vi "SimulatoreStep.vi"() -> ()   [LabVIEW 2019]
doc: "Simulatore Step dei Test:\n\n1. Seleziona la postazione con la data di partenza (opzionale)\n2. Seleziona il Test che vuoi eseguire\n3. Avvia la simulazione e verifica il successo degli Step"
uses:
  ByteGSAPIBase/ByteGSAPIBase.lvclass
  TypeDef/StepSimulationInfo.ctl
  TypeDef/ProcessStatus.ctl
  TypeDef/SimulatoreStates.ctl
  ByteGSAPIBase/TypeDef/Step.ctl
  ByteGSAPIBase/TypeDef/Asset.ctl
  ByteGSAPIBase/TypeDef/Test.ctl
  <vilib>/numeric/Random Number (Range) U64.vi
  <vilib>/numeric/sub_Random U32.vi
panel:
  out "Title":string
  out "Status Control":T2
  out "Waveform Chart":cluster{"Time Elapsed":dbl, dbl}(graph)
  out "Step Info List":T3[](array[typedef])
  in  "Step simulation":bool
  out "Infos":string
  in  "Inizia Test":bool
  in  "Select Test":i32(ring) items=["Test Endurance"=35, "Test Endurance"=36, "Test su Statore H100 dia 65"=29, "Test su Statore H100 dia 65"=31, "Test Endurance"=34, "Test su Statore H100 dia 65"=30, "Effettuare prova sul banco Labview su campione ABC"=40, "Test doppio carico per freni 50Nm/12rpm"=26, "Test su Statore H100 dia 65"=27, "Test su Statore H100 dia 65"=28, "Test su Statore H100 dia 65"=32]
  in  "ByteGSAPIBase in":refnum<class "ByteGSAPIBase.lvclass">
  in  "Exit":bool
  in  "Home":bool
  in  "Ottieni Test Per Postazione":bool
  in  "Starting Date":timestamp format="%<%x>T"
  in  "Workstation":enum16{"POST 1"}(ring)
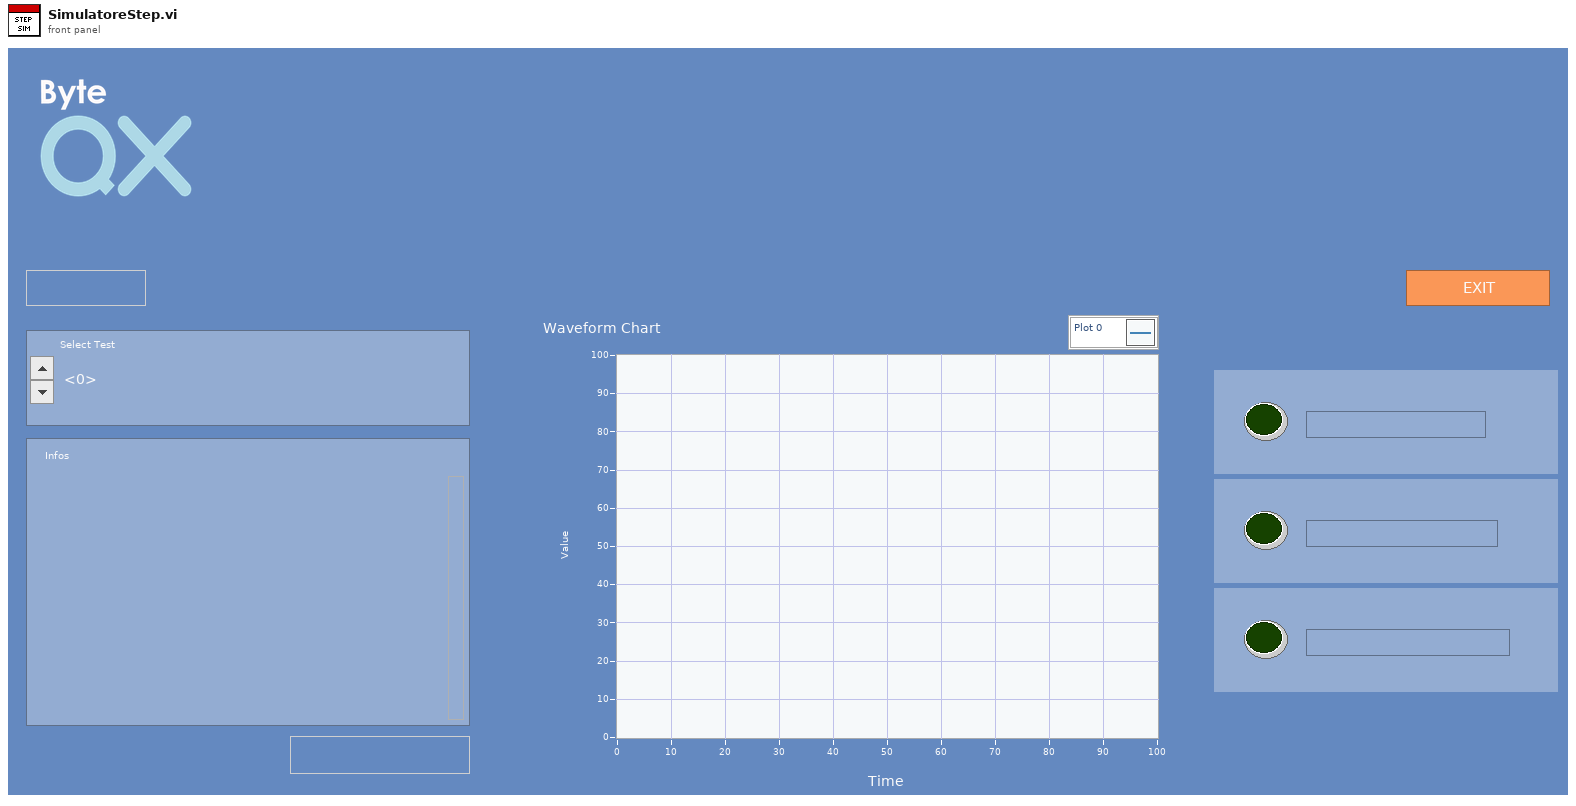
[diagram p1: front panel]
types:
  T1 = typedef "ProcessStatus.ctl" = cluster{"Active":bool, "Process":string}
  T2 = cluster{"Cluster":T1, "Cluster 2":T1, "Cluster 3":T1}
  T3 = typedef "StepSimulationInfo.ctl" = cluster{"Description":string, "Value":dbl, "Outcome":string, "Time Elapsed":dbl, "id":dbl, "Color Box":u32}
  T4 = typedef "SimulatoreStates.ctl" = enum16{"Initialize", "Idle", "GetLimsTestsForBench", "GetLimsTestSteps", "Simulation Start", "WaitForLigths"}
  T5 = typedef "ByteGSWebAPI.lvlib/ByteGSAPIBase.lvclass/Test.ctl" = cluster{"titolo":string, "descrizione":string, "statoprova":string, "assets":T6[], "id":i32, "data_apertura_prova":timestamp}
  T6 = typedef "ByteGSWebAPI.lvlib/ByteGSAPIBase.lvclass/Asset.ctl" = cluster{"descrizione":string, "slug":string, "id":i32}
  T7 = typedef "ByteGSWebAPI.lvlib/ByteGSAPIBase.lvclass/Step.ctl" = cluster{"id":i32, "descrizione":string, "prova":string, "assets":T6[], "criterio_accettazione":string, "valore_criterio_accettazione_max":dbl, "valore_criterio_accettazione_min":dbl, "udm_criterio_accettazione":string, "duration_prova":string, "udm_duration_prova":string, "valore_prova":dbl, "ordine":i32, "user":i32, "link_automation":string, "instruction_automation":string, "data_completamento_checklist":timestamp, "outcome":bool}
  T8 = cluster{"ByteGSAPIBase in":refnum<class "ByteGSAPIBase.lvclass">, "Array dei Test":T5[], "Steps Array":T7[], "Step Info List":T3[], "index":i32, "Previus":T4, "Infos":string, "State":T4, "Status Control":cluster{"Cluster":T1, "Cluster 2":T1, "Cluster 3":T1}, "light position":i32}
  T9 = cluster{"Workstation":refnum<vi>, "Starting Date":refnum<vi>, "Ottieni Test Per Postazione":refnum<vi>, "Infos":refnum<vi>, "Inizia Test":refnum<vi>, "Select Test":refnum<vi>, "Step Info List":refnum<vi>, "Step simulation":refnum<vi>, "Waveform Chart":refnum<vi>, "Status Control":refnum<vi>, "Title":refnum<vi>}
  T10 = enum8{"Enabled", "Disabled", "Disabled and Grayed Out"}
  T11 = cluster{"Workstation":enum16{"POST 1"}, "Starting Date":timestamp, "Select Test":i32}
  T12 = typedef "ByteGSWebAPI.lvlib/ByteGSAPIBase.lvclass/UpdateLimsTestStepData.ctl" = cluster{"outcome":bool, "data_completamento_checklist":timestamp, "udm_duration_prova":string, "valore_prova":dbl, "link_automation":string, "instruction_automation":string, "duration_prova":string}
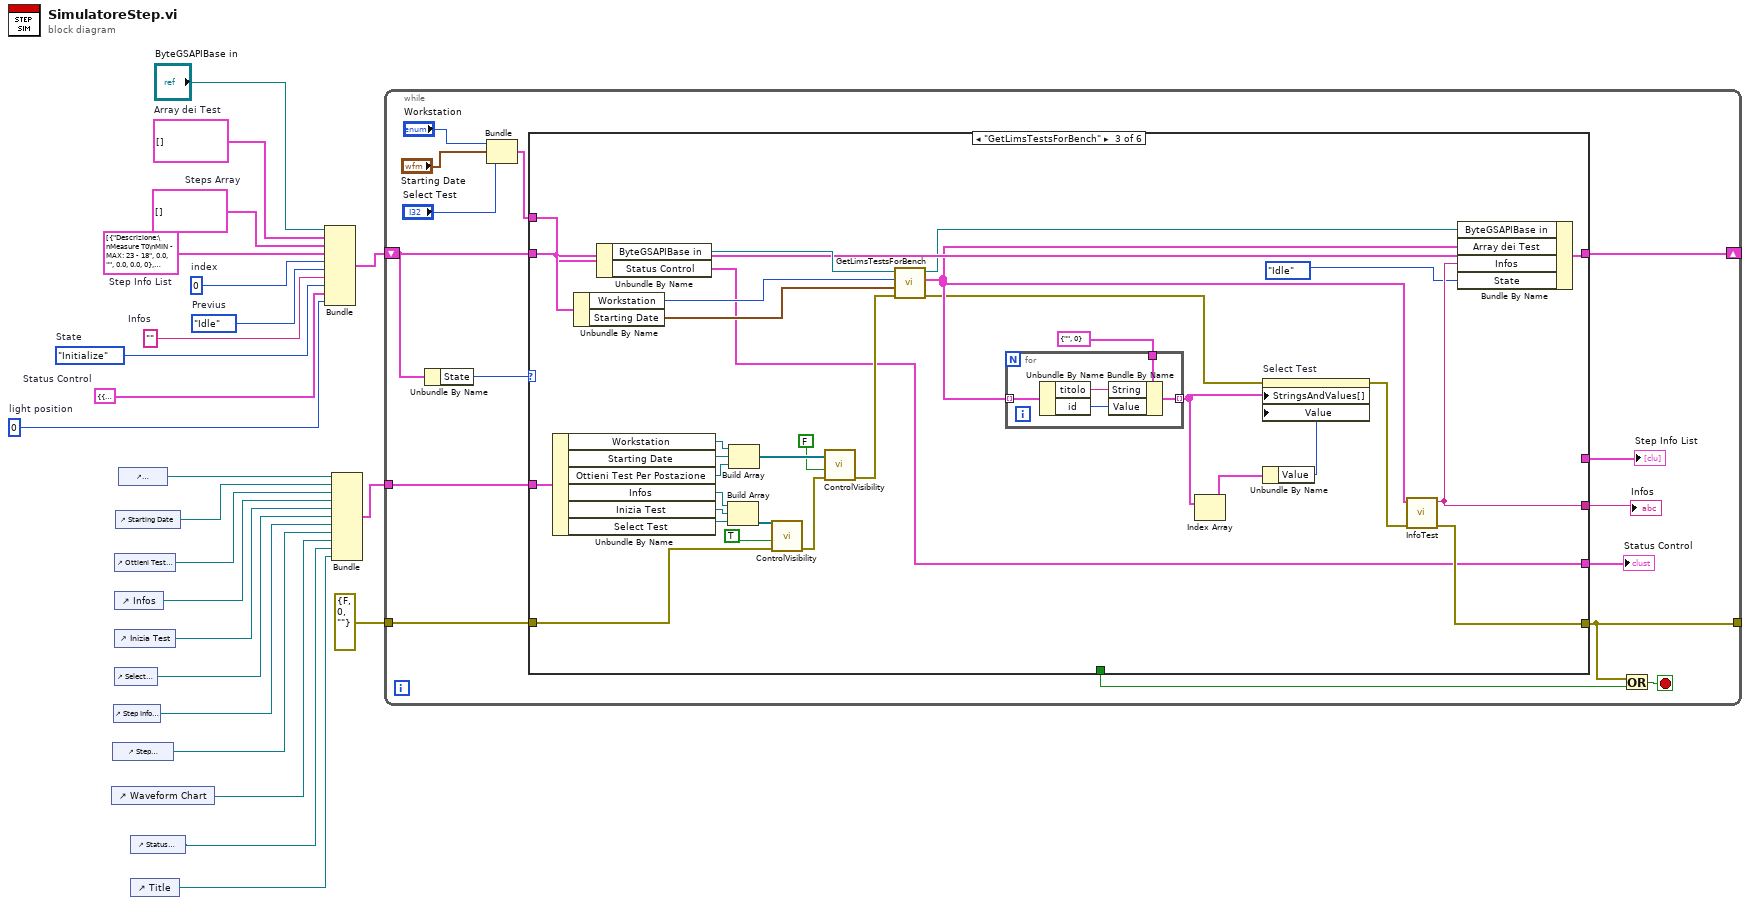
[diagram p0: block diagram]
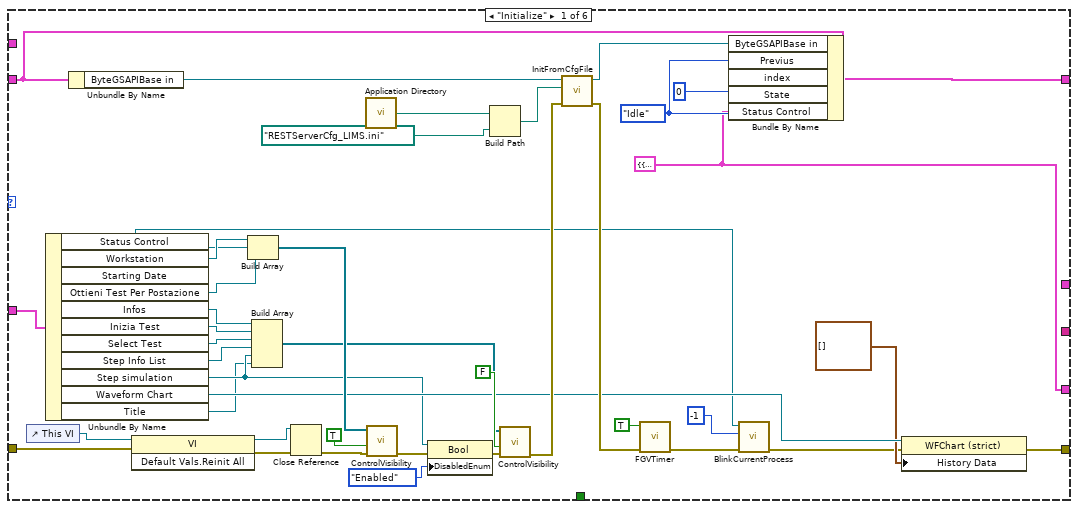
[diagram p2: hidden frame]
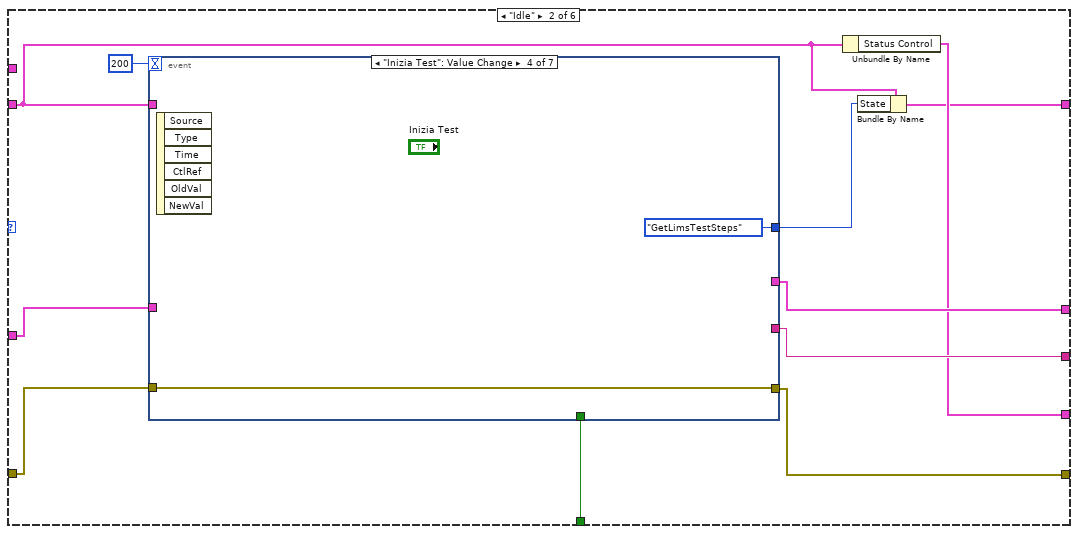
[diagram p3: hidden frame]
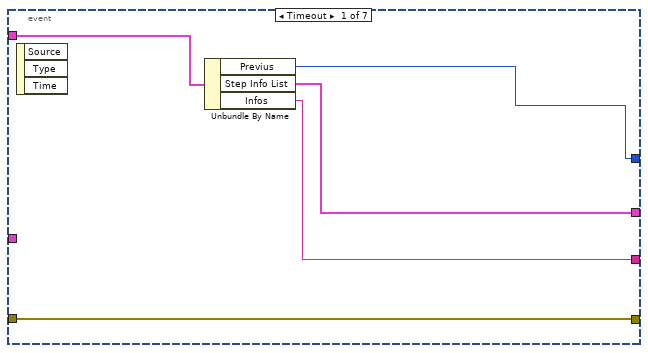
[diagram p4: hidden frame]
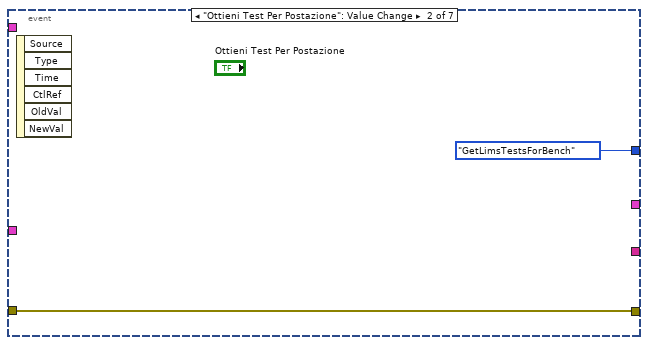
[diagram p5: hidden frame]
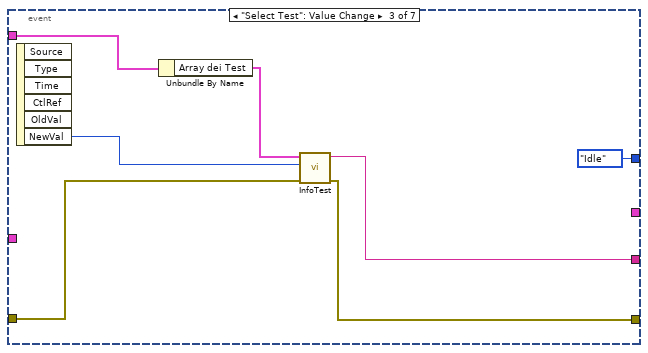
[diagram p6: hidden frame]
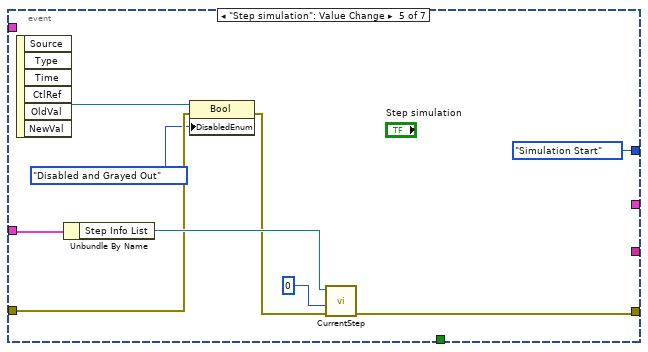
[diagram p7: hidden frame]
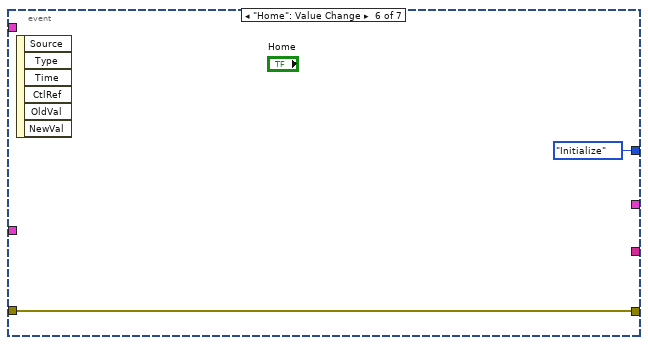
[diagram p8: hidden frame]
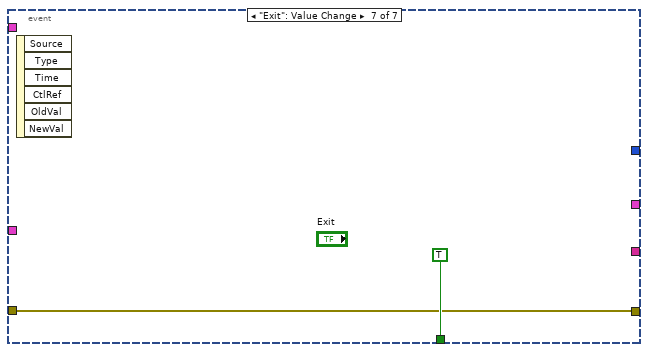
[diagram p9: hidden frame]
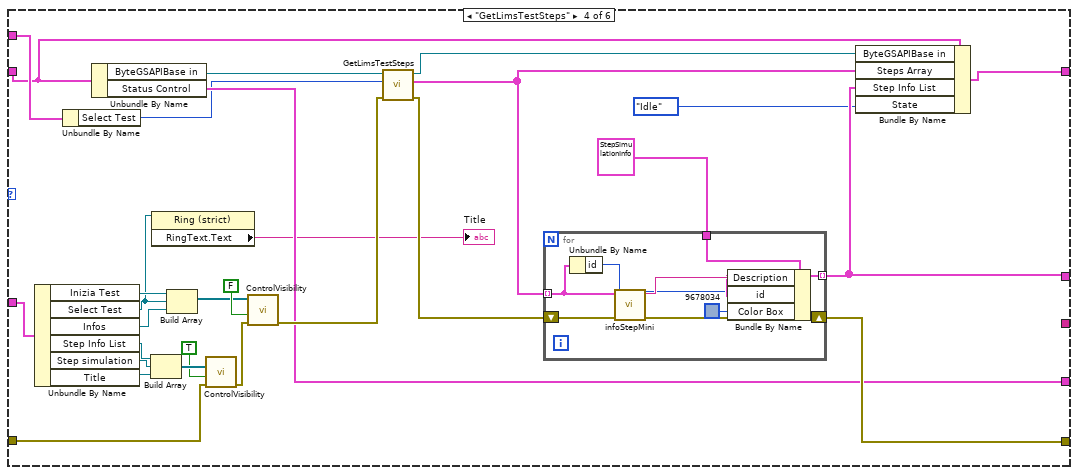
[diagram p10: hidden frame]
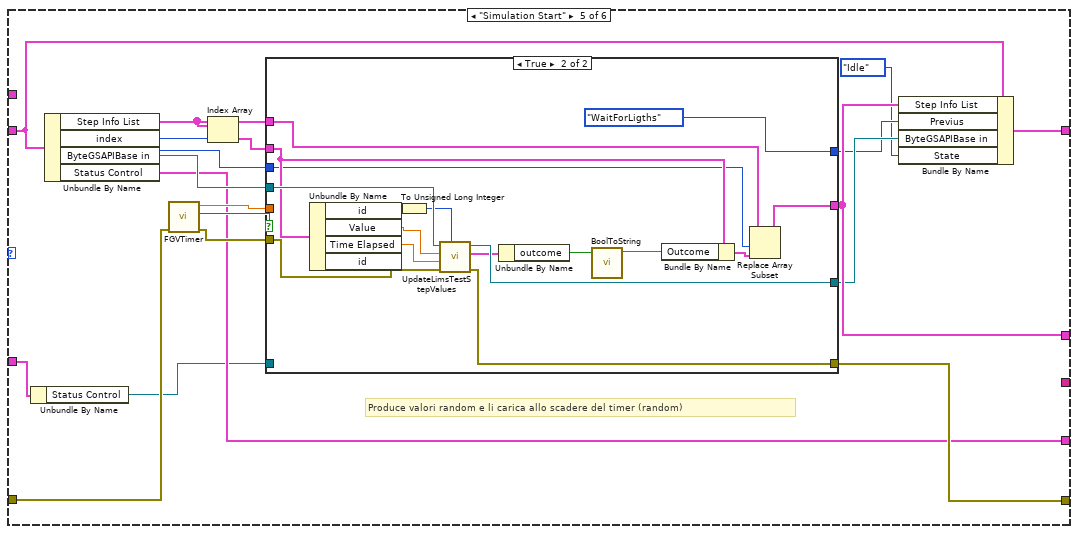
[diagram p11: hidden frame]
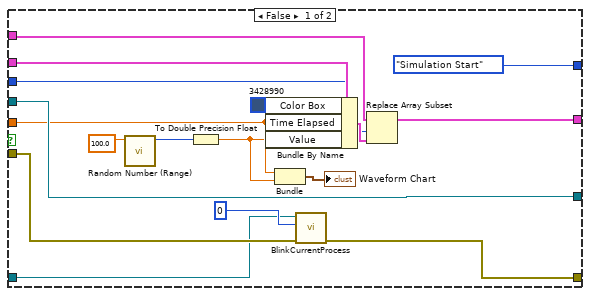
[diagram p12: hidden frame]
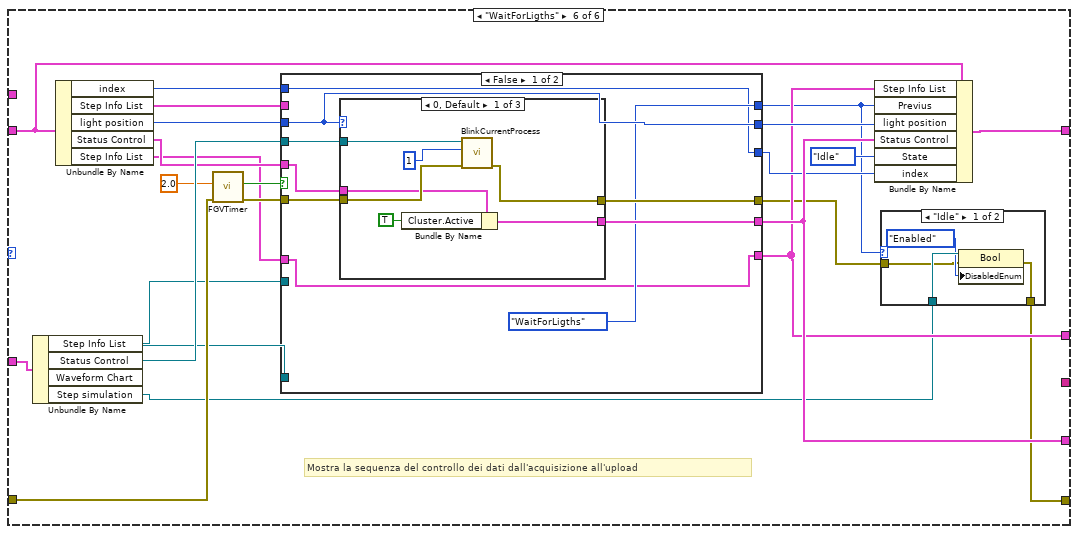
[diagram p13: hidden frame]
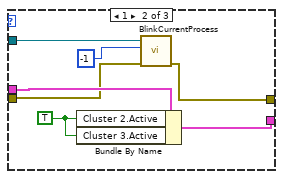
[diagram p15: hidden frame]
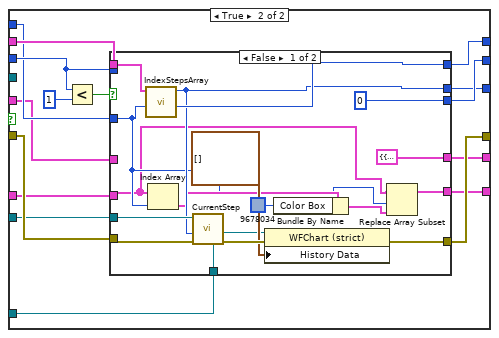
[diagram p17: hidden frame]
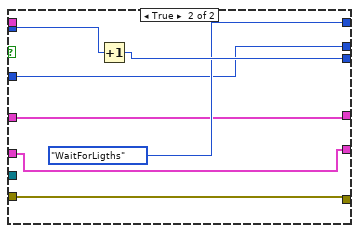
[diagram p18: hidden frame]
diagram:
  w5 = 0  # light position
  w6 = T2 {"Cluster"={"Active"=FALSE, "Process"="Acquisizione Dati"}, "Cluster 2"={"Active"=FALSE, "Process"="Upload Dati"}, "Cluster 3"={"Active"=FALSE, "Process"="Upload Completato"}}  # Status Control
  w9 = ""  # Infos
  w10 = SimulatoreStates."Idle"  # Previus
  w11 = 0  # index
  w12 = T3[] [{"Description"="Descrizione:\nMeasure T0\nMIN - MAX: 23 - 18", "Value"=0.0, "Outcome"="", "Time Elapsed"=0.0, "id"=0.0, "Color Box"=0}, {"Description"="Descrizione:\nSet Nominsl Torque\nMIN - MAX: 1 - -1", "Value"=0.0, "Outcome"="", "Time Elapsed"=0.0, "id"=0.0, "Color Box"=0}, {"Description"="Descrizione:\nVibrazione X,Y,Z\nMIN - MAX: 0 - 0", "Value"=0.0, "Outcome"="", "Time Elapsed"=0.0, "id"=0.0, "Color Box"=0}, {"Description"="Descrizione:\nPlace Motor on the bench. Plug wires on terminal block.\nMIN - MAX: 0 - 0", "Value"=0.0, "Outcome"="", "Time Elapsed"=0.0, "id"=0.0, "Color Box"=0}, {"Description"="Descrizione:\nMeasure R01\nMIN - MAX: 0 - 0", "Value"=0.0, "Outcome"="", "Time Elapsed"=0.0, "id"=0.0, "Color Box"=0}, {"Description"="Descrizione:\nMeasure R02\nMIN - MAX: 0 - 0", "Value"=0.0, "Outcome"="", "Time Elapsed"=0.0, "id"=0.0, "Color Box"=0}]  # Step Info List
  w19 = T5[] []  # Array dei Test
  w18 = T7[] []  # Steps Array
  w8 = SimulatoreStates."Initialize"  # State
  n1 = control-ref of="Waveform Chart"() -> (w3:refnum<vi>)
  n2 = control-ref of="Step simulation"() -> (w13:refnum<vi>)
  n3 = control-ref of="Step Info List"() -> (w4:refnum<vi>)
  n4 = control-ref of="Ottieni Test Per Postazione"() -> (w22:refnum<vi>)
  n5 = control-ref of="Infos"() -> (w16:refnum<vi>)
  n6 = control-ref of="Inizia Test"() -> (w15:refnum<vi>)
  n7 = control-ref of="Select Test"() -> (w14:refnum<vi>)
  n8 = control-ref of="Starting Date"() -> (w23:refnum<vi>)
  n9 = control-ref of="Workstation"() -> (w24:refnum<vi>)
  n10 = control-ref of="Status Control"() -> (w2:refnum<vi>)
  n11 = control-ref of="Title"() -> (w1:refnum<vi>)
  n12 = Bundle("ByteGSAPIBase in"="ByteGSAPIBase in", "Array dei Test"=w19, "Steps Array"=w18, "Step Info List"=w12, "index"=w11, "Previus"=w10, "Infos"=w9, "State"=w8, "Status Control"=w6, "light position"=w5) -> (w17:T8)  [unwired: 1 in]
  n13 = Bundle("Workstation"=w24, "Starting Date"=w23, "Ottieni Test Per Postazione"=w22, "Infos"=w16, "Inizia Test"=w15, "Select Test"=w14, "Step Info List"=w4, "Step simulation"=w13, "Waveform Chart"=w3, "Status Control"=w2, "Title"=w1) -> (w21:T9)  [unwired: 1 in]
  n14 = while {
    tunnel: w21 -> [w35]
    shift-right: [w34] -> _
    shift-left: w17 -> [w28]
    tunnel: errorcluster {"status"=FALSE, "code"=0, "source"=""} ("error in (no error)") -> [w39]
    tunnel: [w31] -> _
    stop <- w30 stop-if-true
    n15 = Unbundle By Name(w28) -> ("State"=w27:T4)
    n16 = Bundle("Workstation"="Workstation", "Starting Date"="Starting Date", "Select Test"="Select Test") -> (w36:T11)  [unwired: 1 in]
    n17 = case shown="\"GetLimsTestsForBench\"" w27 {
      tunnel: w39 -> [w80 w92 w147 w170 w211 w266]
      tunnel: w36 -> [_ _ w152 w186 _ _]
      tunnel: w35 -> [w77 w86 w142 w180 w198 w268]
      tunnel: [w52 w90 w132 w174 w200 w248] -> w31
      tunnel: w28 -> [w65 w83 w151 w183 w208 w263]
      tunnel: [w64 w82 w149 w182 w204 w262] -> w34
      tunnel: [_ w91 w127 _ _ _] -> w32
      tunnel: [_ w88 _ w166 w205 w252] -> w26
      tunnel: [_ w87 _ _ _ _] -> w29
      tunnel: [w46 w84 w123 w163 w196 w260] -> w25
      frame "Initialize" {
        w46 = T2 {"Cluster"={"Active"=FALSE, "Process"="DATA AQUISITION"}, "Cluster 2"={"Active"=FALSE, "Process"="DATA UPLOAD"}, "Cluster 3"={"Active"=FALSE, "Process"="LOADING NEXT STEP"}} ("Status Control")
        w53 = SimulatoreStates."Idle"
        n18 = control-ref of="This VI"() -> (w81:refnum<vi>)
        n19 = Unbundle By Name(w77) -> ("Status Control"=w45:refnum<vi>, "Workstation"=w76:refnum<vi>, "Starting Date"=w75:refnum<vi>, "Ottieni Test Per Postazione"=w74:refnum<vi>, "Infos"=w61:refnum<vi>, "Inizia Test"=w60:refnum<vi>, "Select Test"=w59:refnum<vi>, "Step Info List"=w57:refnum<vi>, "Step simulation"=w42:refnum<vi>, "Waveform Chart"=w51:refnum<vi>, "Title"=w40:refnum<vi>)
        n20 = Unbundle By Name(w65) -> ("ByteGSAPIBase in"=w66:refnum<class "ByteGSAPIBase.lvclass">)
        n21 = invoke class="VI" method="Default Vals.Reinit All"(reference=w81, error in=w80) -> (reference out=w79:refnum<vi>, error out=w78:errorcluster)  [unwired: 1 in, 1 out]
        n22 = Build Array(w76, w75, w74) -> (w73:refnum<vi>[])
        n23 = Build Array(w61, w60, w59, w57, w42, w40) -> (w58:refnum<vi>[])
        n24 = Close Reference(reference=w79, error in (no error)=w78) -> (error out=w72:errorcluster)
        n25 = call <vilib>:"Application Directory.vi"() -> ("Application Directory"=w69:path)
        n26 = call "ControlVisibility.vi"("error in (no error)"=w72, "Visible"=TRUE, "Controls"=w73) -> ("error out"=w44:errorcluster)  [unwired: 8 in]
        n27 = property class="Bool"(reference=w42, error in=w44, "DisabledEnum"=T10."Enabled" ("Disabled")) -> (error out=w43:errorcluster)  [unwired: 1 out]
        n28 = Build Path(base path=w69, name or relative path=path "RESTServerCfg_LIMS.ini") -> (appended path=w70:path)
        n29 = call "ControlVisibility.vi"("error in (no error)"=w43, "Visible"=FALSE, "Controls"=w58) -> ("error out"=w63:errorcluster)  [unwired: 8 in]
        n30 = call-dynamic "InitFromCfgFile.vi"("error in (no error)"=w63, "configuration file path"=w70, "ByteGSAPIBase in"=w66) -> ("error out"=w56:errorcluster, "ByteGSAPIBase out"=w67:refnum<class "ByteGSAPIBase.lvclass">)  [unwired: 7 in]
        n31 = call "FGVTimer.vi"("error in"=w56, "Reset"=TRUE) -> ("error out"=w49:errorcluster)  [unwired: 7 in, 2 out]
        n32 = Bundle By Name(cluster=w65, "ByteGSAPIBase in"=w67, "Previus"=w53, "index"=0, "State"=w53, "Status Control"=w46) -> (w64:T8)
        n33 = call "BlinkCurrentProcess.vi"("error in (no error)"=w49, "index"=-1, "Status Control"=w45) -> ("error out"=w48:errorcluster)  [unwired: 8 in]
        n34 = property class="WFChart (strict)"(reference=w51, error in=w48, "History Data"=cluster{"Time Elapsed":dbl, dbl}[] []) -> (error out=w52:errorcluster)  [unwired: 1 out]
      }
      frame "Idle" {
        n35 = event shown="[3] \"Inizia Test\": Value Change" {
          selector: _ -> [_ _ _ _ _ _ _]
          dyn-events: _ -> [_ _ _ _ _ _ _]
          timeout: 200 -> [_ _ _ _ _ _ _]
          tunnel: [w93 SimulatoreStates."GetLimsTestsForBench" SimulatoreStates."Idle" SimulatoreStates."GetLimsTestSteps" SimulatoreStates."Simulation Start" SimulatoreStates."Initialize" _] -> w85
          tunnel: [w95 _ w104 _ _ _ _] -> w91
          tunnel: w92 -> [w94 w98 w103 w107 w111 w118 w120]
          tunnel: [w94 w98 w102 w107 w115 w118 w120] -> w90
          tunnel: w83 -> [w97 _ w101 _ _ _ _]
          tunnel: [w96 _ _ _ _ _ _] -> w88
          tunnel: [_ _ _ _ _ _ TRUE] -> w87
          tunnel: w86 -> [_ _ _ _ w116 _ _]
          event Timeout {
            n36 = event-data() -> ()  [unwired: 1 in, 3 out]
            n37 = Unbundle By Name(w97) -> ("Previus"=w93:T4, "Step Info List"=w96:T3[], "Infos"=w95:string)
          }
          event "Ottieni Test Per Postazione": Value Change {
            n38 = event-data() -> ()  [unwired: 1 in, 6 out]
          }
          event "Select Test": Value Change {
            n39 = event-data() -> ("NewVal"=w100:i32)  [unwired: 1 in, 5 out]
            n40 = Unbundle By Name(w101) -> ("Array dei Test"=w105:T5[])
            n41 = call "InfoTest.vi"("error in"=w103, "Seleziona Test"=w100, "TestForBenchArray"=w105) -> ("error out"=w102:errorcluster, "Info Test"=w104:string)  [unwired: 7 in]
          }
          event "Inizia Test": Value Change {
            n42 = event-data() -> ()  [unwired: 1 in, 6 out]
          }
          event "Step simulation": Value Change {
            n43 = event-data() -> ("CtlRef"=w112:refnum<vi>)  [unwired: 1 in, 5 out]
            n44 = Unbundle By Name(w116) -> ("Step Info List"=w113:refnum<vi>)
            n45 = property class="Bool"(reference=w112, error in=w111, "DisabledEnum"=T10."Disabled and Grayed Out" ("Disabled")) -> (error out=w110:errorcluster)  [unwired: 1 out]
            n46 = call "CurrentStep.vi"("error in (no error)"=w110, "index"=0, "Array in"=w113) -> ("error out"=w115:errorcluster)  [unwired: 8 in]
          }
          event "Home": Value Change {
            n47 = event-data() -> ()  [unwired: 1 in, 6 out]
          }
          event "Exit": Value Change {
            n48 = event-data() -> ()  [unwired: 1 in, 6 out]
          }
        }
        n49 = Unbundle By Name(w83) -> ("Status Control"=w84:T2)
        n50 = Bundle By Name(cluster=w83, "State"=w85) -> (w82:T8)
      }
      frame "GetLimsTestsForBench" {
        n51 = Unbundle By Name(w142) -> ("Workstation"=w141:refnum<vi>, "Starting Date"=w140:refnum<vi>, "Ottieni Test Per Postazione"=w139:refnum<vi>, "Infos"=w138:refnum<vi>, "Inizia Test"=w137:refnum<vi>, "Select Test"=w136:refnum<vi>)
        n52 = Unbundle By Name(w152) -> ("Workstation"=w126:enum16{"POST 1"}, "Starting Date"=w125:timestamp)
        n53 = Unbundle By Name(w151) -> ("ByteGSAPIBase in"=w153:refnum<class "ByteGSAPIBase.lvclass">, "Status Control"=w123:T2)
        n54 = Build Array(w138, w137, w136) -> (w130:refnum<vi>[])
        n55 = Build Array(w141, w140, w139) -> (w131:refnum<vi>[])
        n56 = call "ControlVisibility.vi"("error in (no error)"=w147, "Visible"=TRUE, "Controls"=w130) -> ("error out"=w135:errorcluster)  [unwired: 8 in]
        n57 = call "ControlVisibility.vi"("error in (no error)"=w135, "Visible"=FALSE, "Controls"=w131) -> ("error out"=w134:errorcluster)  [unwired: 8 in]
        n58 = call-dynamic "GetLimsTestsForBench.vi"("error in (no error)"=w134, "Data Partenza"=w125, "Postazione"=w126, "ByteGSAPIBase in"=w153) -> ("error out"=w122:errorcluster, "Tests for bench"=w143:T5[], "ByteGSAPIBase out"=w150:refnum<class "ByteGSAPIBase.lvclass">)  [unwired: 5 in]
        n59 = for {
          tunnel: w143 -> [w158] mode=indexing
          tunnel: [w155] -> w146 mode=indexing
          tunnel: cluster{"String":string, "Value":u16} {"String"="", "Value"=0} ("Cluster") -> [w154]
          n60 = Unbundle By Name(w158) -> ("titolo"=w157:string, "id"=w156:i32)
          n61 = Bundle By Name(cluster=w154, "String"=w157, "Value"=w156) -> (w155:cluster{"String":string, "Value":u16})
        }
        n62 = Index Array(array=w146) -> (element=w145:cluster{"String":string, "Value":u16})  [unwired: 1 in]
        n63 = Unbundle By Name(w145) -> ("Value"=w144:u16)
        n64 = property on="Select Test" class="Ring (strict)"(error in=w122, "StringsAndValues[]"=w146, "Value"=w144) -> (error out=w133:errorcluster)  [unwired: 1 in, 1 out]
        n65 = call "InfoTest.vi"("error in"=w133, "TestForBenchArray"=w143) -> ("error out"=w132:errorcluster, "Info Test"=w127:string)  [unwired: 8 in]
        n66 = Bundle By Name(cluster=w151, "ByteGSAPIBase in"=w150, "Array dei Test"=w143, "Infos"=w127, "State"=SimulatoreStates."Idle") -> (w149:T8)
      }
      frame "GetLimsTestSteps" {
        n67 = Unbundle By Name(w180) -> ("Inizia Test"=w179:refnum<vi>, "Select Test"=w161:refnum<vi>, "Infos"=w173:refnum<vi>, "Step Info List"=w172:refnum<vi>, "Step simulation"=w167:refnum<vi>, "Title"=w162:refnum<vi>)
        n68 = Unbundle By Name(w186) -> ("Select Test"=w160:i32)
        n69 = Unbundle By Name(w183) -> ("ByteGSAPIBase in"=w185:refnum<class "ByteGSAPIBase.lvclass">, "Status Control"=w163:T2)
        n70 = Build Array(w172, w167, w162) -> (w171:refnum<vi>[])
        n71 = property class="Ring (strict)"(reference=w161) -> ("RingText.Text"=→"Title":string)  [unwired: 1 in, 2 out]
        n72 = Build Array(w179, w161, w173) -> (w178:refnum<vi>[])
        n73 = call "ControlVisibility.vi"("error in (no error)"=w170, "Visible"=TRUE, "Controls"=w171) -> ("error out"=w169:errorcluster)  [unwired: 8 in]
        n74 = call "ControlVisibility.vi"("error in (no error)"=w169, "Visible"=FALSE, "Controls"=w178) -> ("error out"=w177:errorcluster)  [unwired: 8 in]
        n75 = call-dynamic "GetLimsTestSteps.vi"("error in (no error)"=w177, "Test-id"=w160, "ByteGSAPIBase in"=w185) -> ("error out"=w175:errorcluster, "Test Steps List"=w176:T7[], "ByteGSAPIBase out"=w184:refnum<class "ByteGSAPIBase.lvclass">)  [unwired: 6 in]
        n76 = for {
          tunnel: w176 -> [w189] mode=indexing
          shift-right: [w193] -> w174
          shift-left: w175 -> [w194]
          tunnel: T3 {"Description"="Descrizione:\nMeasure T0\nMIN - MAX: 23 - 18", "Value"=0.0, "Outcome"="", "Time Elapsed"=0.0, "id"=0.0, "Color Box"=0} ("Cluster") -> [w192]
          tunnel: [w190] -> w166 mode=indexing
          n77 = Unbundle By Name(w189) -> ("id"=w188:i32)
          n78 = call "infoStepMini.vi"("error in (no error)"=w194, "StepList"=w189) -> ("error out"=w193:errorcluster, "Info Test"=w191:string)  [unwired: 8 in]
          n79 = Bundle By Name(cluster=w192, "Description"=w191, "id"=w188, "Color Box"=u32 9678034) -> (w190:T3)
        }
        n80 = Bundle By Name(cluster=w183, "ByteGSAPIBase in"=w184, "Steps Array"=w176, "Step Info List"=w166, "State"=SimulatoreStates."Idle") -> (w182:T8)
      }
      frame "Simulation Start" {
        # "Produce valori random e li carica allo scadere del timer (random)"
        n81 = Unbundle By Name(w198) -> ("Status Control"=w195:refnum<vi>)
        n82 = Unbundle By Name(w208) -> ("Step Info List"=w207:T3[], "index"=w206:i32, "ByteGSAPIBase in"=w203:refnum<class "ByteGSAPIBase.lvclass">, "Status Control"=w196:T2)
        n83 = call "FGVTimer.vi"("error in"=w211) -> ("error out"=w202:errorcluster, "Elapsed?"=w212:bool, "Time Elapsed"=w209:dbl)  [unwired: 8 in]
        n84 = Index Array(array=w207, index=w206) -> (element=w210:T3)
        n85 = case shown="True" w212 {
          tunnel: w210 -> [w229 w243]
          tunnel: w209 -> [w220 _]
          tunnel: w207 -> [w227 w237]
          tunnel: w206 -> [w221 w238]
          tunnel: [w225 w246] -> w205
          tunnel: w203 -> [w224 w244]
          tunnel: w202 -> [w218 w234]
          tunnel: [w224 w240] -> w201
          tunnel: [w217 w232] -> w200
          tunnel: [SimulatoreStates."Simulation Start" ("Previus") SimulatoreStates."WaitForLigths" ("Previus")] -> w199
          tunnel: w195 -> [w213 _]
          frame False {
            n86 = call-poly <vilib>:"Random Number (Range).vi"("upper bound (100)"=100.0) -> ("number"=w222:u64)  [unwired: 10 in]
            n87 = To Double Precision Float(number=w222) -> (double precision float=w219:dbl)
            n88 = Bundle By Name(cluster=w229, "Color Box"=u32 3428990, "Time Elapsed"=w220, "Value"=w219) -> (w226:T3)
            n89 = Bundle("Time Elapsed"=w220, w219) -> (→"Waveform Chart":cluster{"Time Elapsed":dbl, dbl})  [unwired: 1 in]
            n90 = call "BlinkCurrentProcess.vi"("error in (no error)"=w218, "index"=0, "Status Control"=w213) -> ("error out"=w217:errorcluster)  [unwired: 8 in]
            n91 = Replace Array Subset(array=w227, new element=w226, index=w221) -> (w225:T3[])
          }
          frame True {
            n92 = Unbundle By Name(w243) -> ("id"=w231:dbl, "Value"=w242:dbl, "Time Elapsed"=w241:dbl)  [unwired: 1 out]
            n93 = To Unsigned Long Integer(number=w231) -> (unsigned 32bit integer=w230:u32)
            n94 = call-dynamic "UpdateLimsTestStepValues.vi"("step_id"=w230, "error in (no error)"=w234, "duration_hours"=w241, "value"=w242, "ByteGSAPIBase in"=w244) -> ("error out"=w232:errorcluster, "Result Step"=w239:T12, "ByteGSAPIBase out"=w240:refnum<class "ByteGSAPIBase.lvclass">)  [unwired: 4 in]
            n95 = Unbundle By Name(w239) -> ("outcome"=w235:bool)
            n96 = call "BoolToString.vi"("outcome"=w235) -> ("String"=w236:string)  [unwired: 10 in]
            n97 = Bundle By Name(cluster=w243, "Outcome"=w236) -> (w245:T3)
            n98 = Replace Array Subset(array=w237, new element=w245, index=w238) -> (w246:T3[])
          }
        }
        n99 = Bundle By Name(cluster=w208, "Step Info List"=w205, "Previus"=w199, "ByteGSAPIBase in"=w201, "State"=SimulatoreStates."Idle") -> (w204:T8)
      }
      frame "WaitForLigths" {
        # "Mostra la sequenza del controllo dei dati dall'acquisizione all'upload"
        n100 = Unbundle By Name(w268) -> ("Step Info List"=w255:refnum<vi>, "Status Control"=w267:refnum<vi>, "Waveform Chart"=w254:refnum<vi>, "Step simulation"=w250:refnum<vi>)
        n101 = Unbundle By Name(w263) -> ("index"=w257:i32, "Step Info List"=w258:T3[], "light position"=w269:i32, "Status Control"=w264:T2, "Step Info List"=w253:T3[])
        n102 = call "FGVTimer.vi"("error in"=w266, "set timer"=2.0) -> ("error out"=w265:errorcluster, "Elapsed?"=w270:bool)  [unwired: 7 in, 1 out]
        n103 = case shown="False" w270 {
          tunnel: w269 -> [w279 w314]
          tunnel: w267 -> [w284 _]
          tunnel: w265 -> [w283 w308]
          tunnel: w264 -> [w282 w303]
          tunnel: [w281 w304] -> w260
          tunnel: [w280 w306] -> w249
          tunnel: [w279 w313] -> w259
          tunnel: [SimulatoreStates."WaitForLigths" ("Previus") w312] -> w251
          tunnel: w258 -> [_ w311]
          tunnel: w257 -> [w277 w310]
          tunnel: [w277 w309] -> w256
          tunnel: w255 -> [_ w307]
          tunnel: w254 -> [_ w305]
          tunnel: w253 -> [w276 w302]
          tunnel: [w276 w301] -> w252
          frame False {
            n104 = case shown="0, Default" w279 {
              tunnel: w284 -> [w285 w292 _]
              tunnel: w283 -> [w290 w296 w299]
              tunnel: w282 -> [w288 w297 w300]
              tunnel: [w287 w295 w300] -> w281
              tunnel: [w286 w294 w299] -> w280
              frame 0, Default {
                n105 = Bundle By Name(cluster=w288, "Cluster.Active"=TRUE) -> (w287:T2)
                n106 = call "BlinkCurrentProcess.vi"("error in (no error)"=w290, "index"=1, "Status Control"=w285) -> ("error out"=w286:errorcluster)  [unwired: 8 in]
              }
              frame 1 {
                w293 = TRUE ("Cluster.Active")
                n107 = Bundle By Name(cluster=w297, "Cluster 2.Active"=w293, "Cluster 3.Active"=w293) -> (w295:T2)
                n108 = call "BlinkCurrentProcess.vi"("error in (no error)"=w296, "index"=-1, "Status Control"=w292) -> ("error out"=w294:errorcluster)  [unwired: 8 in]
              }
              frame 2 {
              }
            }
          }
          frame True {
            n109 = Less?(x=w314, y=1) -> (x < y?=w315:bool)
            n110 = case shown="False" w315 {
              tunnel: w314 -> [_ w340]
              tunnel: [0 w339] -> w313
              tunnel: [w332 SimulatoreStates."WaitForLigths" ("Previus")] -> w312
              tunnel: w311 -> [w331 _]
              tunnel: w310 -> [w320 w337]
              tunnel: [w324 w337] -> w309
              tunnel: w308 -> [w330 w336]
              tunnel: w307 -> [w329 _]
              tunnel: [w326 w336] -> w306
              tunnel: w305 -> [w325 _]
              tunnel: [T2 {"Cluster"={"Active"=FALSE, "Process"="DATA AQUISITION"}, "Cluster 2"={"Active"=FALSE, "Process"="DATA UPLOAD"}, "Cluster 3"={"Active"=FALSE, "Process"="LOADING NEXT STEP"}} ("Status Control") w335] -> w304
              tunnel: w303 -> [_ w335]
              tunnel: w302 -> [w319 w334]
              tunnel: [w318 w334] -> w301
              frame False {
                n111 = call "IndexStepsArray.vi"("index"=w320, "Steps Array"=w331) -> ("Previus"=w332:T4, "Index out"=w324:i32)  [unwired: 8 in]
                n112 = Index Array(array=w319, index=w320) -> (element=w323:T3)
                n113 = call "CurrentStep.vi"("error in (no error)"=w330, "index"=w324, "Array in"=w329) -> ("error out"=w328:errorcluster)  [unwired: 8 in]
                n114 = property class="WFChart (strict)"(reference=w325, error in=w328, "History Data"=cluster{"Time Elapsed":dbl, dbl}[] []) -> (error out=w326:errorcluster)  [unwired: 1 out]
                n115 = Bundle By Name(cluster=w323, "Color Box"=u32 9678034) -> (w321:T3)
                n116 = Replace Array Subset(array=w319, new element=w321, index=w320) -> (w318:T3[])
              }
              frame True {
                n117 = Increment(x=w340) -> (x+1=w339:i32)
              }
            }
          }
        }
        n118 = Bundle By Name(cluster=w263, "Step Info List"=w252, "Previus"=w251, "light position"=w259, "Status Control"=w260, "State"=SimulatoreStates."Idle", "index"=w256) -> (w262:T8)
        n119 = case shown="\"Idle\"" w251 {
          tunnel: w250 -> [w274 _]
          tunnel: w249 -> [w272 w275]
          tunnel: [w271 w275] -> w248
          frame "Idle" {
            n120 = property class="Bool"(reference=w274, error in=w272, "DisabledEnum"=T10."Enabled" ("Disabled")) -> (error out=w271:errorcluster)  [unwired: 1 out]
          }
          frame Default {
          }
        }
      }
    }
    "Infos" <- w32
    "Step Info List" <- w26
    "Status Control" <- w25
    n121 = Or(x=w31, y=w29) -> (x .or. y?=w30:bool)
  }
